vi "PathDrawerMain.vi"() -> ()   [LabVIEW 2020]
uses:
  StartingPositions.ctl
  Dawgma Programming Library/Controls/PurePursuit/PathFileData.ctl
  Dawgma Programming Library/Controls/PurePursuit/RobotNeededPathData.ctl
  <vilib>/Utility/miscctls.llb/LVBoundsTypeDef.ctl
  Robot Project/Configuration/Constants.vi
panel:
  out "Test Inch Coordinates":cluster{dbl, dbl}[](array[cluster])=[{289.544235924933, 135.50670241286863}, {0.0, -0.0}, {328.92225201072387, 121.60857908847186}, {215.42091152815016, 204.99731903485255}, {283.75335120643433, 155.1957104557641}]
  out "value":T1[](array[typedef])=[{"RobotNeeded"={"Path"=[{289.544235924933, 127.39946380697052}, {287.98440012511463, 121.65498051124526}, {286.41922502031144, 115.91988239594286}, {284.8425468097273, 110.20506726948979}, {283.24633395018986, 104.52472200513712}, {281.61937943101464, 98.89861870378402}, {279.9454878089578, 93.35531222737507}, {278.2008591447135, 87.93676042855766}, {276.35024133935286, 82.70511682939853}, {274.3412254828133, 77.75279489984473}, {272.09576087008793, 73.21743176567836}, {269.4975173972782, 69.30417285758647}, {266.3730504540402, 66.31888533561163}, {262.30977093522324, 64.13267492925793}, {257.6170022887625, 62.48225945252617}, {252.50215191030858, 61.19110326109334}, {247.10429046762434, 60.14083593442563}, {241.5166672476604, 59.252088190224804}, {235.8018071548225, 58.471641965553985}, {230.0016338079975, 57.763814107212845}, {224.14425732034206, 57.10467874503091}, {218.2485291335668, 56.478193499430674}, {212.3270758147521, 55.87360015253457}, {206.38842308808773, 55.2836904580848}, {200.43813908174548, 54.70361642727725}, {194.4802433054481, 54.13015590178437}, {188.51708827270537, 53.56111165140166}, {182.55050868849642, 52.99504342054156}, {176.58171996706054, 52.430973067035474}, {170.6114588037997, 51.86824641350337}, {164.6402875329216, 51.306429540500694}, {158.66867548195333, 50.74523633232348}, {152.69698950924862, 50.184482181742624}, {146.72554975069153, 49.62405174097509}, {140.7547236952346, 49.06388019791822}, {134.785000977592, 48.50394578938929}, {128.8170560229984, 47.94426701710933}, {122.8518418626467, 47.38490492824676}, {116.89074159778129, 46.82596881662714}, {110.93580758402727, 46.26763838286973}, {104.99009019888962, 45.7101898480154}, {99.05814276927747, 45.15404369729131}, {93.14674575066984, 44.599832973624785}, {87.26600325213306, 44.04850237548434}, {81.4309817746881, 43.50146179439437}, {75.6641490637674, 42.96081623768789}, {69.99901263505986, 42.429706416458394}, {64.48554690731844, 41.91281674321665}, {59.198284254035755, 41.4171340541128}, {54.24838019418854, 40.953079037223475}, {49.80160857908847, 40.53619302949062}], "MaxVel"=150.0, "MaxAccel"=150.0, "Backwards?"=TRUE, "PointSpacing"=6.0, "LookaheadDist"=17.0, "Speed/Curve"=3.0, "SlowDistanceAtEnd"=0.0, "SlowSpeed"=15.0, "MaxDeAccel"=120.0}, "Meta"={"Path (px)"=[{351, 192}, {336, 249}, {144, 267}], "RobotWidth"=31.5, "RobotLength"=38.5, "CenterOfRotYOffset"=17.0, "Roundedness"=0.8606565656565657, "StartingPositionPreset"=5, "PathName"=""}}, {"RobotNeeded"={"Path"=[{41.694369973190355, 41.694369973190355}, {47.64761218323431, 40.94676925259769}, {53.60085959538599, 40.19914995082028}, {59.554106695902426, 39.451516891020106}, {65.50734952417288, 38.70387941982743}, {71.46058708655964, 37.956246193008944}, {77.41382093064641, 37.2086221311749}, {83.36705361599451, 36.461007989713714}, {89.32028708212145, 35.71340175224902}, {95.27352165286956, 34.96580062830542}, {101.22675591339359, 34.21820267296435}, {107.17998723937053, 33.4706075949886}, {113.13321251833818, 32.723016842705846}, {119.08642860902965, 31.975433361115666}, {125.03963222056859, 31.227861451959267}, {130.99281926364412, 30.480307293161797}, {136.94598341959534, 29.732778542763988}, {142.89911342764645, 28.985292503880892}, {148.8521970948602, 28.237856543424133}, {154.80519717572702, 27.490525695688227}, {160.7580926557246, 26.743311754896478}, {166.7108090144928, 25.996307137451996}, {172.66326246213927, 25.249610988717894}, {178.61533307346468, 24.50335830315379}, {184.56682545232815, 23.757776428670198}, {190.51745097236886, 23.013204152377078}, {196.46678999980696, 22.270130566274368}, {202.4142158693123, 21.529284158414665}, {208.35878682551095, 20.79176138061672}, {214.29909655137962, 20.05920100132194}, {220.23305131995286, 19.334042109666537}, {226.15753100580926, 18.619918062154806}, {232.06788077313638, 17.92224896220281}, {237.95715568369013, 17.249121917891284}, {243.81499755234879, 16.61260080269244}, {249.62595906000692, 16.030669585531108}, {255.36700689486312, 15.530167782478935}, {261.0037825664052, 15.151071217352833}, {266.48505855860725, 14.953090658917299}, {271.7344114271029, 15.025170414334722}, {276.6378873606053, 15.500037107436073}, {281.02552281994616, 16.5756320859188}, {284.64383847846, 18.547123872167777}, {287.2812495218884, 21.833836599641202}, {289.2609081448733, 26.00205669815591}, {290.7994717493821, 30.760784058063827}, {292.04218375653704, 35.914613439968605}, {293.0863889218551, 41.33211000782484}, {293.9972923578865, 46.924534979681674}, {294.8185166544407, 52.63147263946088}, {295.5791655320445, 58.411043001053216}, {296.2985359831856, 64.23312215031287}, {296.9892418555871, 70.074469274851}, {297.6592556133157, 75.91496594399388}, {298.3131992777047, 81.73435754239064}, {298.95309316561156, 87.50897171708034}, {299.57868315910804, 93.20788489320849}, {300.18739942296327, 98.78791642871371}, {300.7739401344564, 104.18663870347694}, {301.32941304122085, 109.31227034681507}, {301.839895859845, 114.02881614064651}, {302.28418230563005, 118.13404825737267}], "MaxVel"=150.0, "MaxAccel"=150.0, "Backwards?"=FALSE, "PointSpacing"=6.0, "LookaheadDist"=17.0, "Speed/Curve"=3.0, "SlowDistanceAtEnd"=0.0, "SlowSpeed"=15.0, "MaxDeAccel"=120.0}, "Meta"={"Path (px)"=[{137, 266}, {352, 293}, {362, 200}], "RobotWidth"=31.5, "RobotLength"=38.5, "CenterOfRotYOffset"=17.0, "Roundedness"=0.8606565656565657, "StartingPositionPreset"=5, "PathName"=""}}] {"RobotNeeded"."SlowSpeed" format="%#_13g"; "RobotNeeded"."SlowDistanceAtEnd" format="%#_13g"; "RobotNeeded"."Speed/Curve" format="%#_13g"}
  in  "NoUpdate":bool
  out "PathsStorage":T1[](array[typedef])=[{"RobotNeeded"={"Path"=[{425.05093833780165, 52.11796246648794}, {430.9905583996291, 52.11796246648794}, {436.9198305935917, 52.11796246648794}, {442.8265331238852, 52.11796246648794}, {448.6941988585669, 52.11796246648794}, {454.50043960617046, 52.11796246648794}, {460.2111611561605, 52.11796246648794}, {465.7769300637667, 52.11796246648794}, {471.1226712041929, 52.11796246648794}, {476.13506368722386, 52.11796246648794}, {480.64343163538877, 52.11796246648794}], "MaxVel"=100.0, "MaxAccel"=150.0, "Backwards?"=FALSE, "PointSpacing"=6.0, "LookaheadDist"=17.0, "Speed/Curve"=3.0, "SlowDistanceAtEnd"=0.0, "SlowSpeed"=15.0, "MaxDeAccel"=120.0}, "Meta"={"Path (px)"=[{468, 257}, {516, 257}], "RobotWidth"=32.0, "RobotLength"=39.0, "CenterOfRotYOffset"=17.0, "Roundedness"=0.8526363636363636, "StartingPositionPreset"=6, "PathName"=""}}] {"RobotNeeded"."SlowSpeed" format="%#_13g"; "RobotNeeded"."SlowDistanceAtEnd" format="%#_13g"; "RobotNeeded"."Speed/Curve" format="%#_13g"}
  in  "Tab Control":enum32{"Path", "Load/Save"}(tab)
  in  "SetStart":bool
  in  "Deaccel":dbl=120.0 format="%#_13g"
  in  "SlowSpeed":dbl=15.0 format="%#_13g"
  in  "SlowDistanceAtEnd":dbl format="%#_13g"
  in  "Speed/Curve":dbl=3.0 format="%#_13g"
  in  "DriveBackwards?":bool
  in  "Lookahead":dbl=17.0
  in  "Points (in)":cluster{dbl, dbl}[](array[cluster])=[{425.05093833780165, 52.11796246648794}, {480.64343163538877, 52.11796246648794}]
  out "Points (px)":cluster{dbl, dbl}[](array[cluster])=[{468.0, 257.0}, {516.0, 257.0}]
  in  "Roundedness":dbl(slide)=0.8526363636363636 scale=0.6..0.997
  in  "PointSpacing":dbl=6.0 min=1.0 format="%#_13g"
  in  "Flip Path":bool
  in  "MaxVel":dbl=100.0 format="%#_13g"
  in  "Accel":dbl=150.0 format="%#_13g"
  in  "StartingPosition":T3=enum."No Preset"
  in  "Multiple Paths":i32(listbox)
  in  "ExportAllToRobot":bool
  in  "LocalTempPaths":i32(listbox)
  out "standard output":string
  in  "SaveToLocal":bool
  in  "LoadFromLocal":bool
  in  "ExportToRobot":bool
  in  "LoadAllFromRobot":bool
  in  "LocalPaths":i32(listbox)
  out "standard error":string="NI Linux Real-Time (run mode)\n\nLog in with your NI-Auth credentials.\n\n"
  in  "LocalFileNames":string[](array[string])=["STARTINGPOSITIONTEST.txt"]
  out "Path Drawer":T4(plugin-control)
  # "(Double Click)"
  # "INSTRUCTIONS"
  # "The red line is the path that the robot recieves. Everything else is to help create that path\n\nUse the multi-line tool to draw a path. Double click to stop drawing.\nHover over a node and press backspace to remove it.\nPress I to insert a new node (at the end of the path only, for now)\n\nUse the contols to input robot width, height, and center of rotation offset,\nHow far apart the points in the \"real world units\" path are,\nWhether the robot travels on the left or right of your green lines, and\nthe roundedness of the path. (Note: point spacing affects roundedness)\n\nYou can manually edit the green node's location in the path with the Points array,\nor drag the nodes on the image\n\nPress Export To File and enter the file name (no extension) to save the path to a file in the\nThisVIsDirectory\\Paths\\ folder\n\nIf you acidentally clear your path press Z quickly to get it back"
  # "Responses of CMDs run"
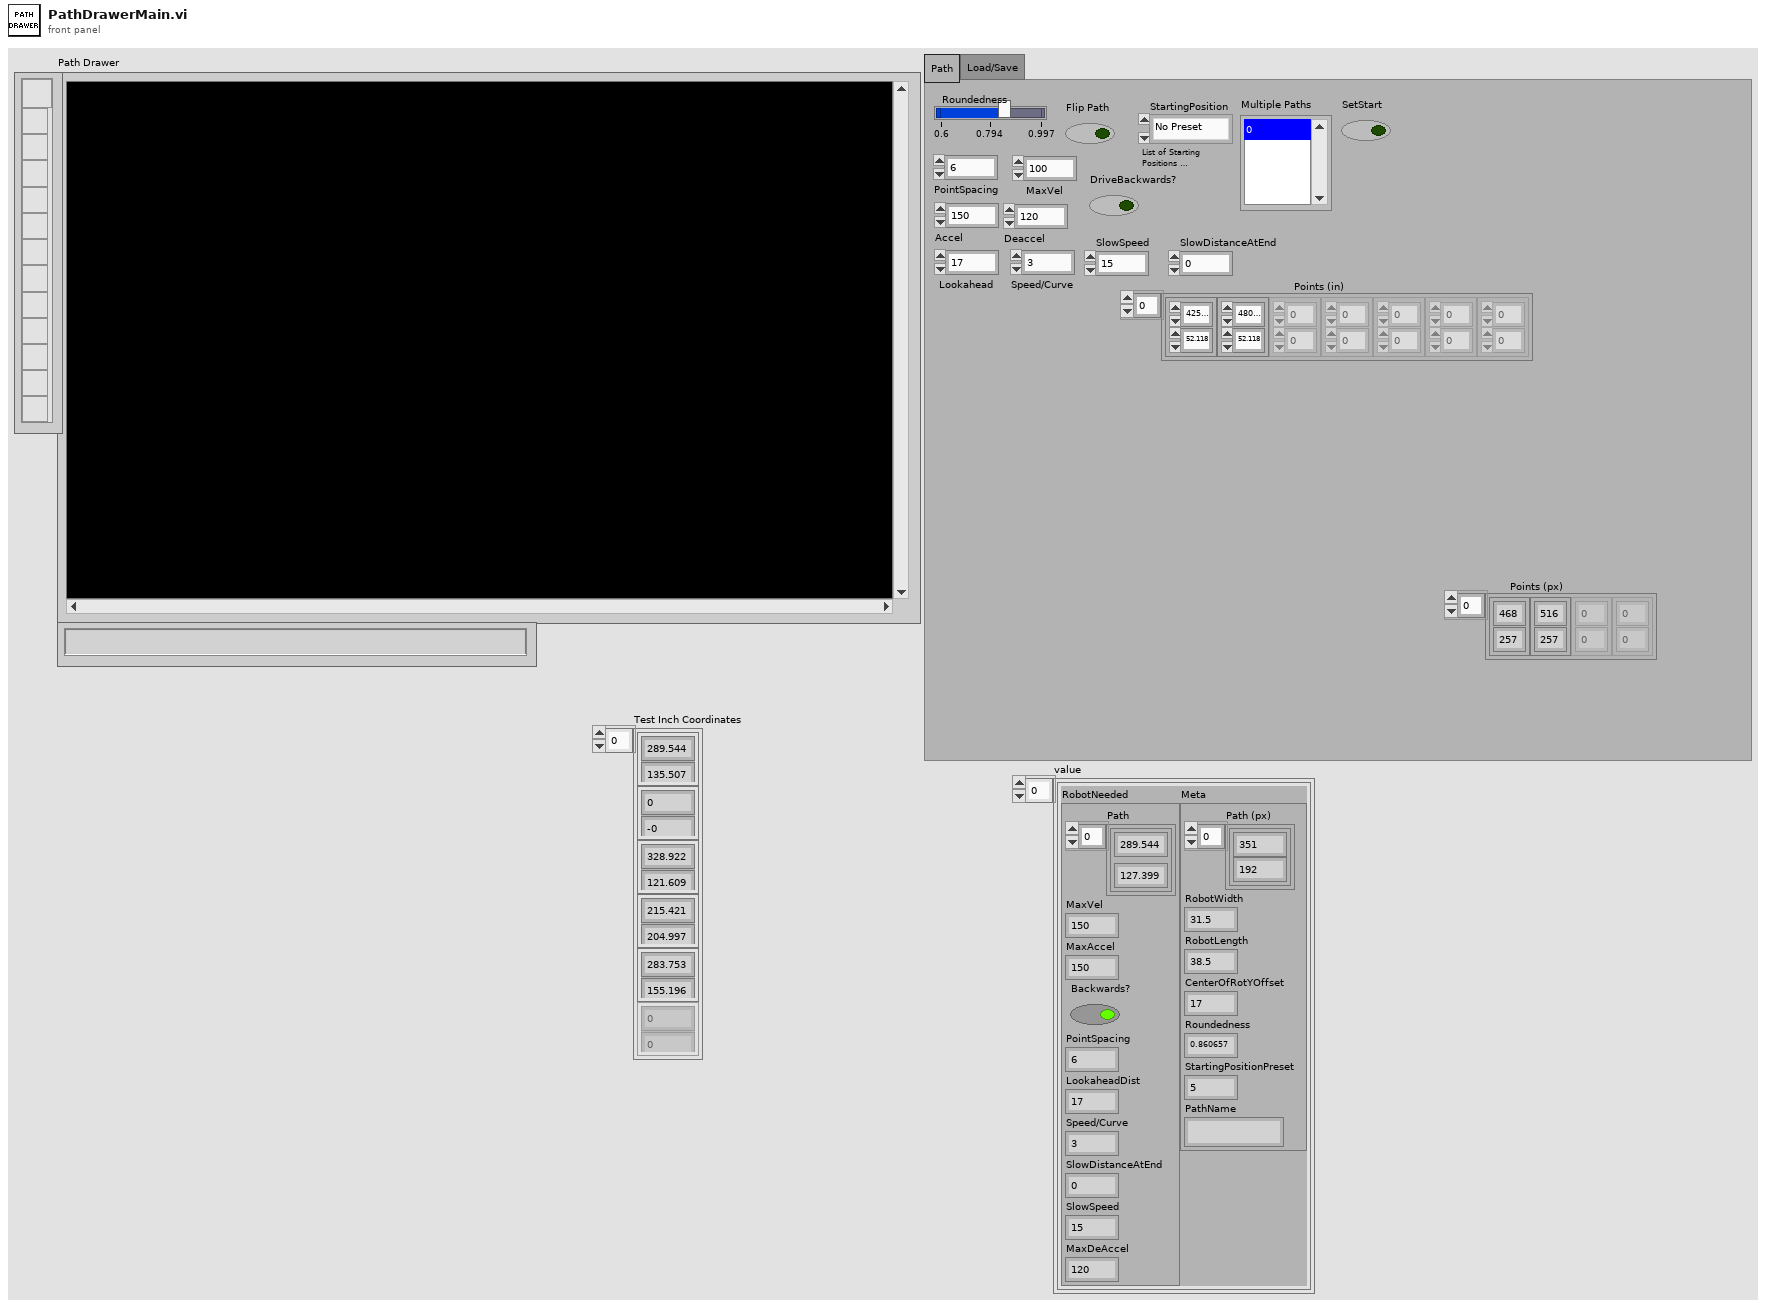
[diagram p1: front panel]
types:
  T1 = typedef "PathFileData.ctl" = cluster{"RobotNeeded":T2, "Meta":cluster{"Path (px)":cluster{i32, i32}[], "RobotWidth":dbl, "RobotLength":dbl, "CenterOfRotYOffset":dbl, "Roundedness":dbl, "StartingPositionPreset":u32, "PathName":string}}
  T2 = typedef "RobotNeededPathData.ctl" = cluster{"Path":cluster{dbl, dbl}[], "MaxVel":dbl, "MaxAccel":dbl, "Backwards?":bool, "PointSpacing":dbl, "LookaheadDist":dbl, "Speed/Curve":dbl, "SlowDistanceAtEnd":dbl, "SlowSpeed":dbl, "MaxDeAccel":dbl}
  T3 = typedef "StartingPositions.ctl" = enum16{"1", "2", "3", "4", "5", "6", "No Preset"}
  T4 = typedef "IMAQ Image.ctl" = refnum<image>
  T5 = typedef "Image Type" = u32
  T6 = enum16{"open", "replace", "create", "open or create", "replace or create", "replace or create with confirmation"}
  T7 = typedef "LVBoundsTypeDef.ctl" = cluster{"Width":u32, "Height":u32}
  T8 = cluster{"Global Rectangle":i32[], "Contours":cluster{"Contour Type":u32, "ROI Type":u32, "Points":i32[]}[]}
  T9 = cluster{"Contour Type":u32, "ROI Type":u32, "Points":i32[]}[]
  T10 = cluster{"Contour Type":u32, "ROI Type":u32, "Points":i32[]}
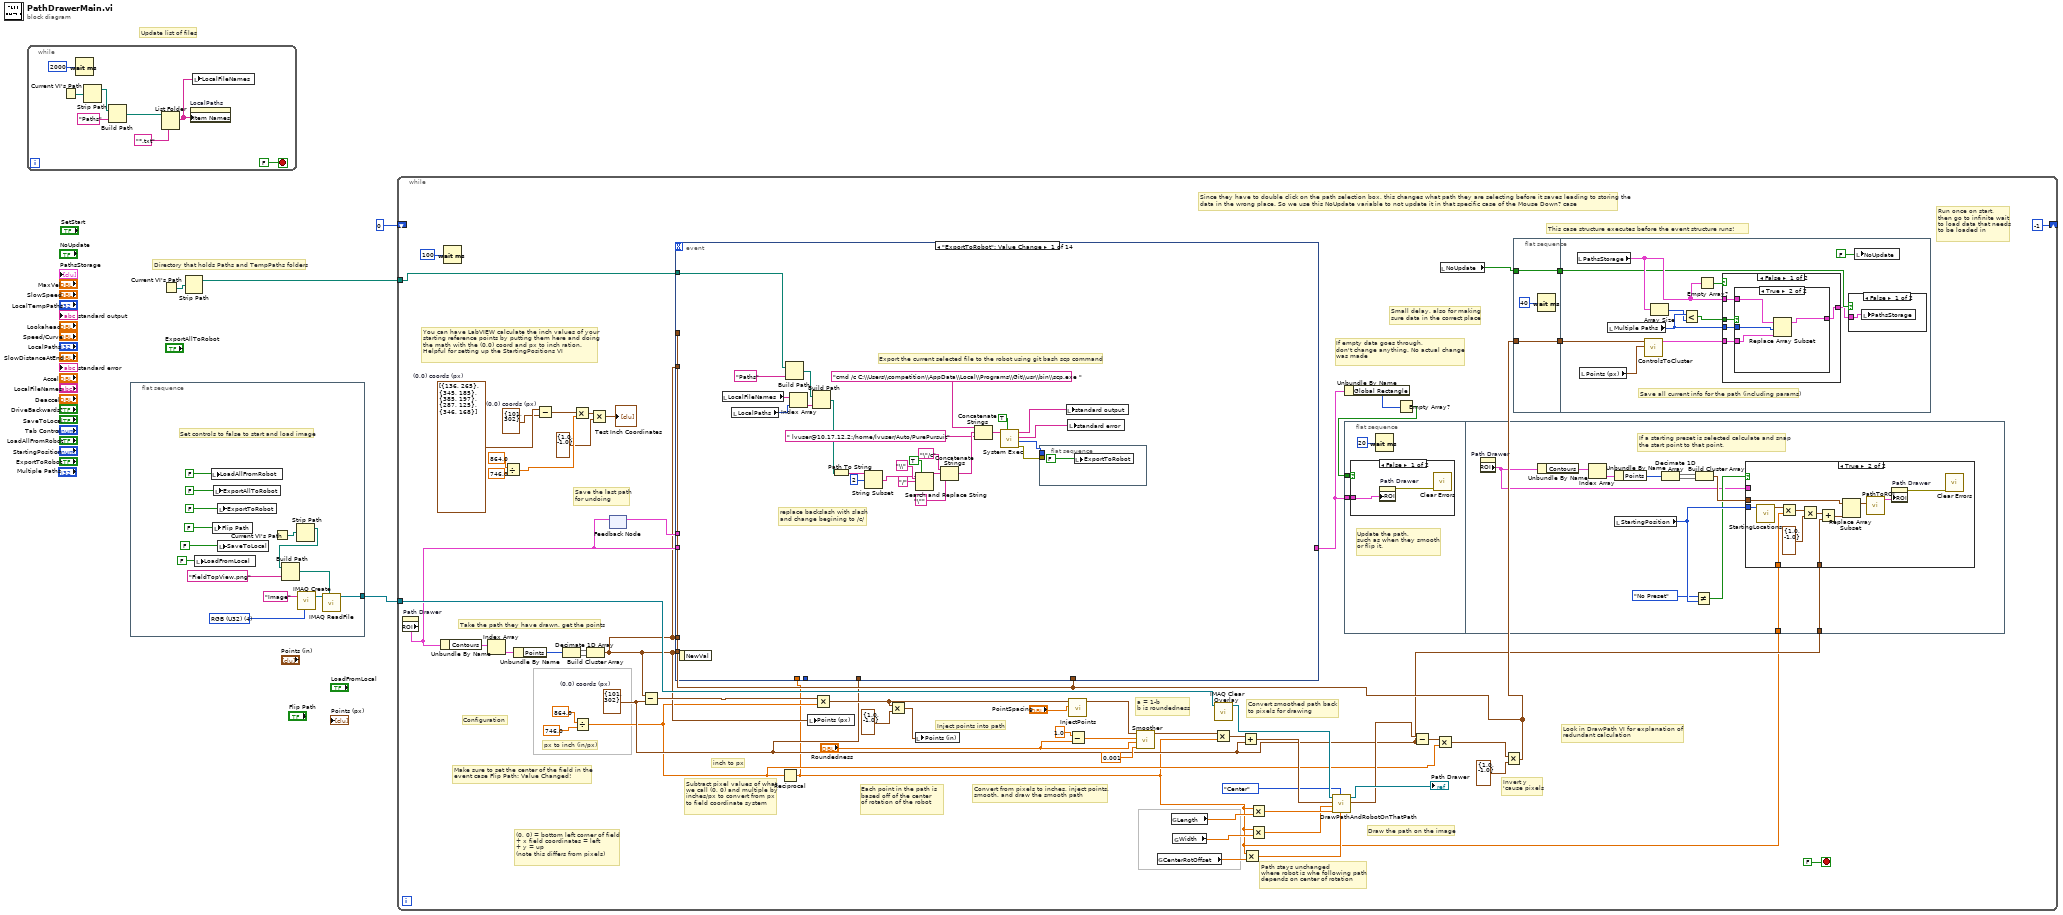
[diagram p0: block diagram]
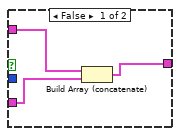
[diagram p3: hidden frame]
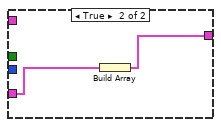
[diagram p4: hidden frame]
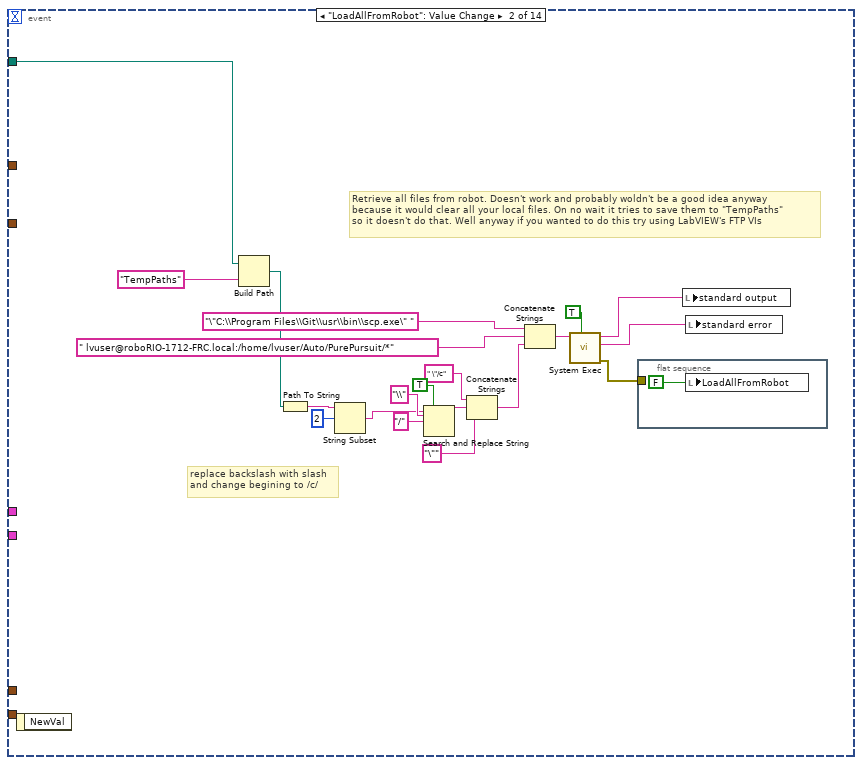
[diagram p7: hidden frame]
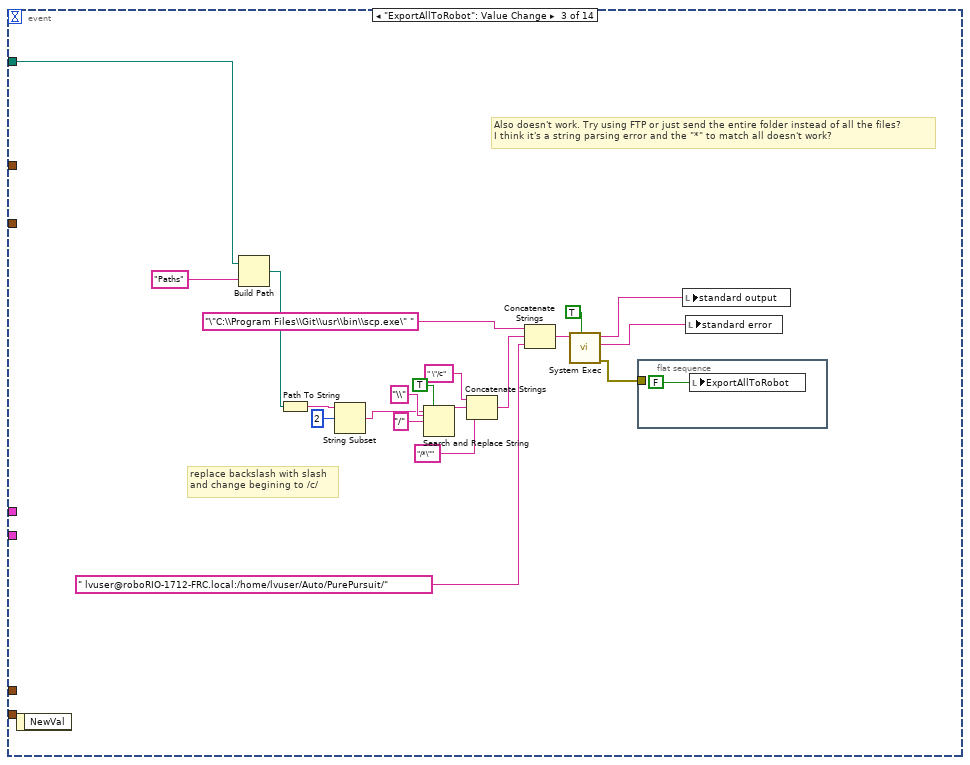
[diagram p8: hidden frame]
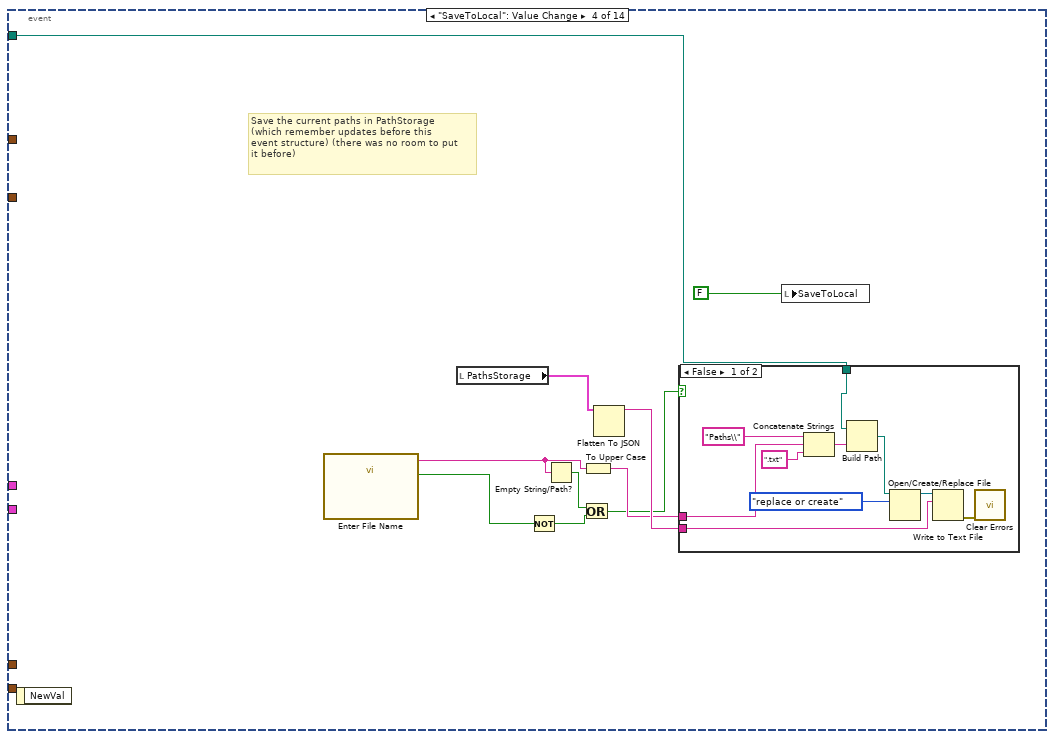
[diagram p9: hidden frame]
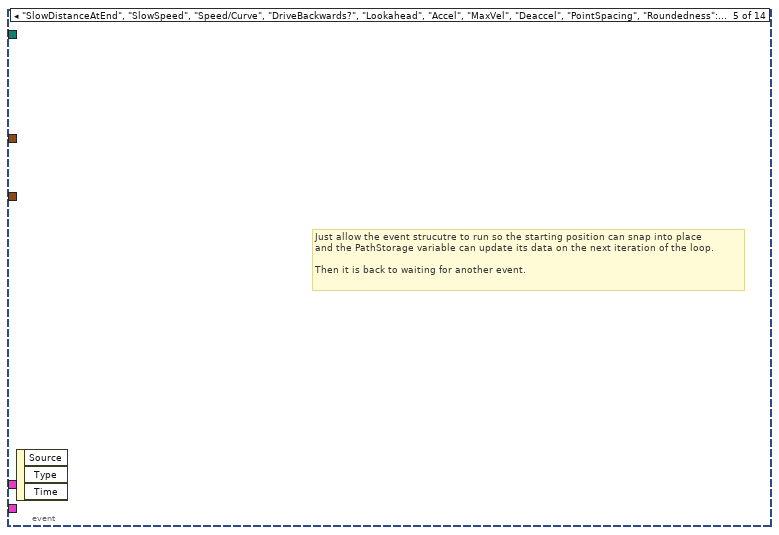
[diagram p11: hidden frame]
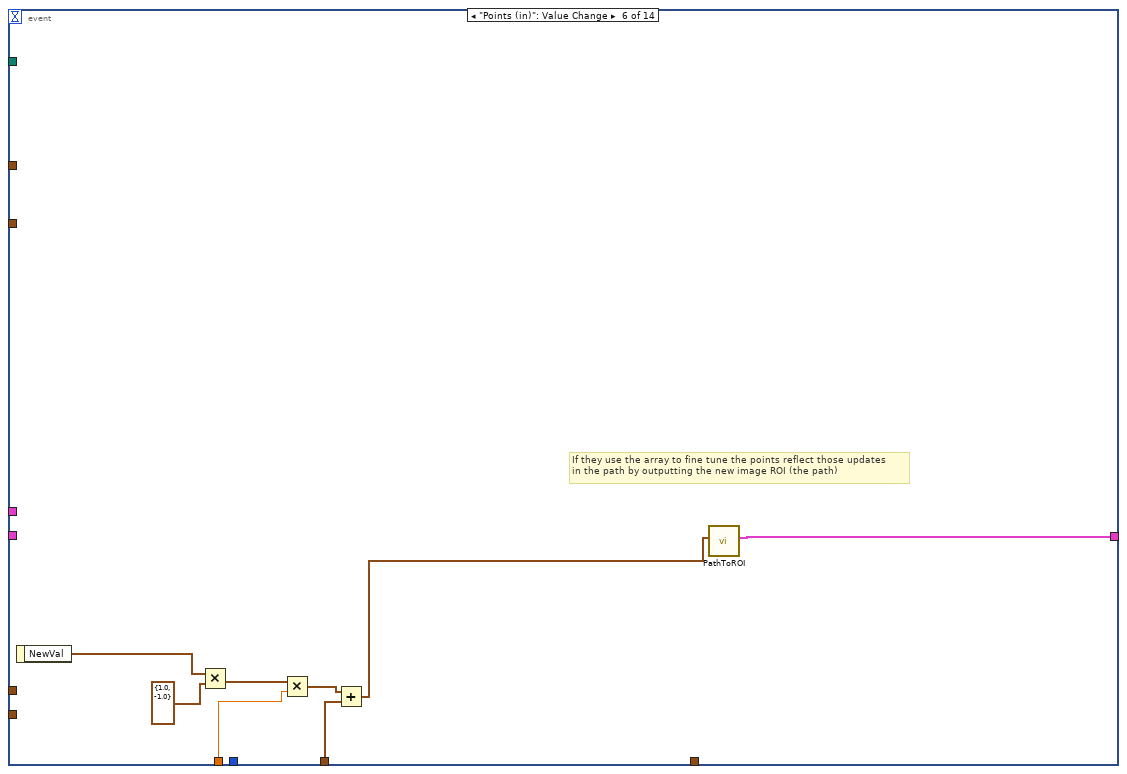
[diagram p12: hidden frame]
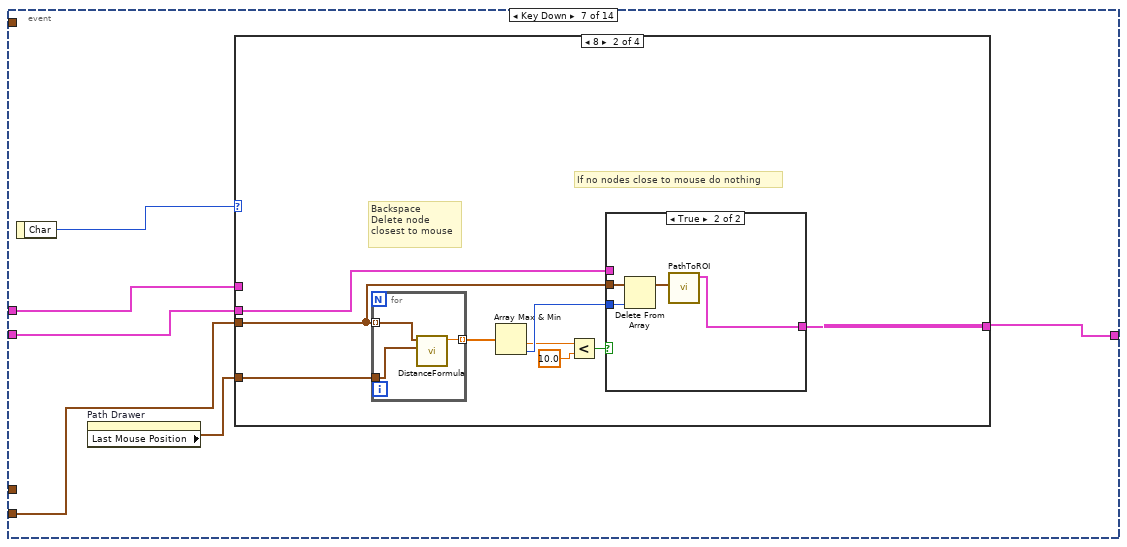
[diagram p13: hidden frame]
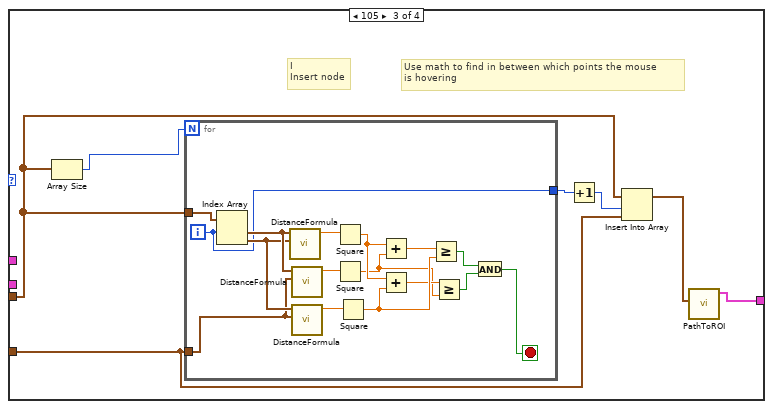
[diagram p16: hidden frame]
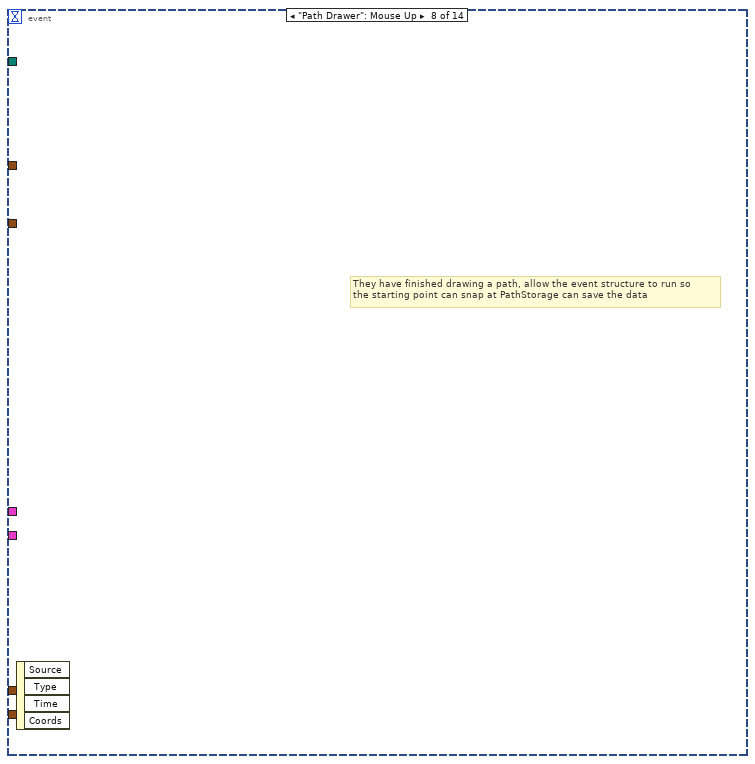
[diagram p18: hidden frame]
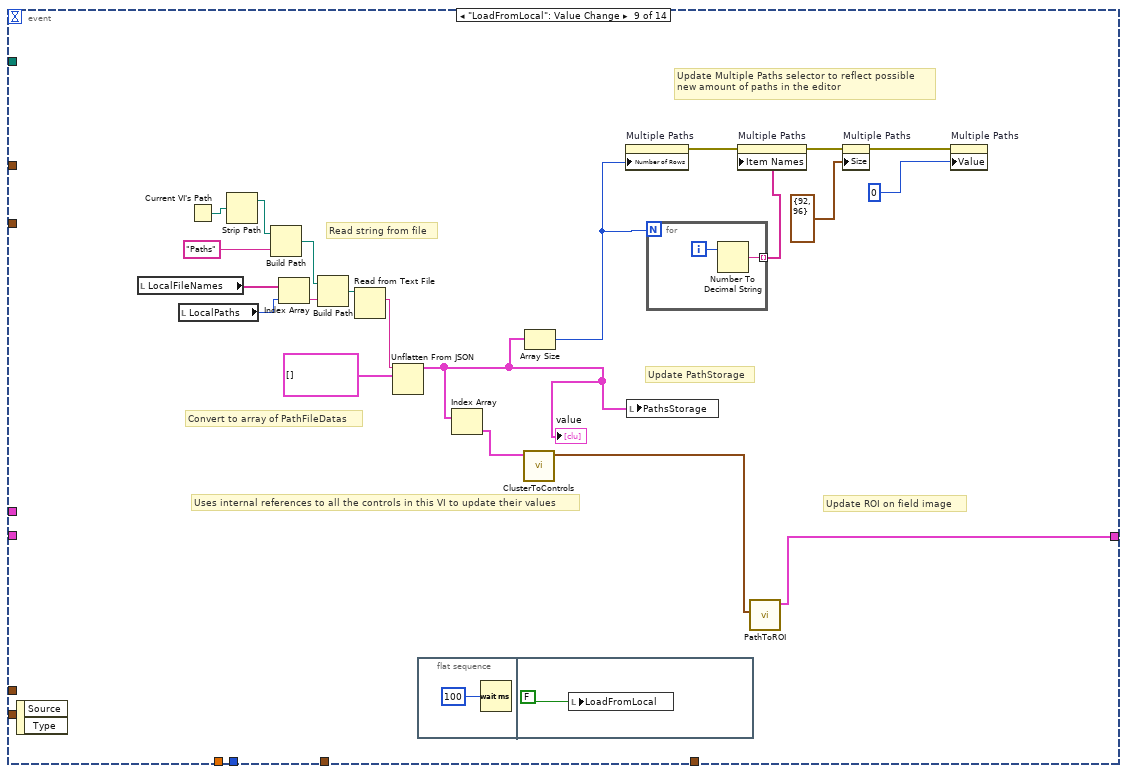
[diagram p19: hidden frame]
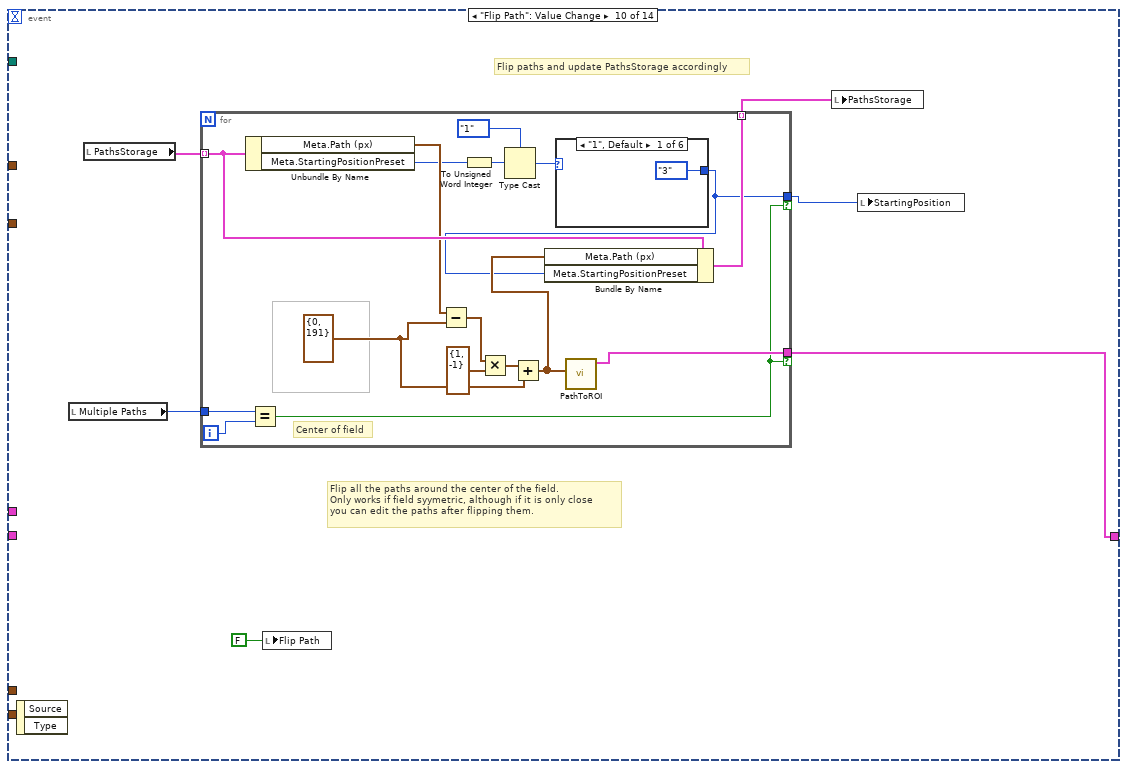
[diagram p20: hidden frame]
diagram:
  # "Update list of files"
  # "Directory that holds Paths and TempPaths folders"
  n1 = while {
    stop <- FALSE stop-if-true
    n2 = Current VI's Path() -> (path=w7:path)
    n3 = Wait (ms)(milliseconds to wait=u32 2000) -> ()  [unwired: 1 out]
    n4 = Strip Path(path=w7) -> (stripped path=w6:path)  [unwired: 1 out]
    n5 = Build Path(base path=w6, name or relative path="Paths") -> (appended path=w9:path)
    n6 = List Folder(path=w9, pattern="*.txt") -> (filenames=w11:string[])  [unwired: 2 in, 3 out]
    n7 = property on="LocalPaths" class="LstBox (strict)"("Item Names"=w11) -> ()  [unwired: 2 in, 2 out]
    n8 = local write "LocalFileNames"(w11) -> ()
  }
  n9 = flat-sequence {
    tunnel: [w21] -> w4
    frame #0 {
      w23 = T5 4 items=["Grayscale (U8)", "Grayscale (I16)", "Grayscale (SGL)", "Complex (CSG)", "RGB (U32)", "HSL (U32)", "RGB (U64)", "Grayscale (U16)"] ("Image Type")
      # "Set controls to false to start and load image"
      n10 = local write "LoadFromLocal"(FALSE ("Export To File")) -> ()
      n11 = local write "LoadAllFromRobot"(FALSE ("Export To File")) -> ()
      n12 = local write "Flip Path"(FALSE ("Export To File")) -> ()
      n13 = local write "ExportAllToRobot"(FALSE ("Export To File")) -> ()
      n14 = local write "ExportToRobot"(FALSE ("Export To File")) -> ()
      n15 = local write "SaveToLocal"(FALSE ("Export To File")) -> ()
      n16 = Current VI's Path() -> (path=w16:path)
      n17 = Strip Path(path=w16) -> (stripped path=w15:path)  [unwired: 1 out]
      n18 = Build Path(base path=w15, name or relative path="FieldTopView.png") -> (appended path=w25:path)
      n19 = call "IMAQ Create"("Image Name"="Image", "Image Type"=w23) -> ("New Image"=w22:T4)  [unwired: 3 in, 1 out]
      n20 = call "IMAQ ReadFile"("File Path"=w25, "Image"=w22) -> ("Image Out"=w21:T4)  [unwired: 5 in, 4 out]
    }
  }
  n21 = Current VI's Path() -> (path=w3:path)
  n22 = Strip Path(path=w3) -> (stripped path=w2:path)  [unwired: 1 out]
  n23 = while {
    tunnel: w4 -> [w80]
    tunnel: w2 -> [w55]
    shift-right: [-1] -> _
    shift-left: 0 -> [_]
    stop <- FALSE stop-if-true
    w27 = cluster{i32, i32} {101, 302}  # (0,0) coords (px)
    w28 = cluster{i32, i32}[] [{136, 265}, {345, 185}, {385, 197}, {287, 125}, {346, 168}]  # (0,0) coords (px)
    w38 = cluster{i32, i32} {101, 302}  # (0,0) coords (px)
    # "Each point in the path is\nbased off of the center\nof rotation of the robot"
    # "You can have LabVIEW calculate the inch values of your\nstarting reference points by putting them here and doing\nthe math with the (0,0) coord and px to inch ration.\nHelpful for setting up the StartingPositions VI"
    # "Small delay, also for making\nsure data in the correct place"
    # "Since they have to double click on the path selection box, this changes what path they are selecting before it saves leading to storing the\ndata in the wrong place. So we use this NoUpdate variable to not update it in that specific case of the Mouse Down? case"
    # "This case structure executes before the event structure runs!"
    # "Look in DrawPath VI for explanation of \nredundant calculation"
    # "Draw the path on the image"
    # "a = 1-b\nb is roundedness"
    # "Inject points into path"
    # "(0, 0) = bottom left corner of field\n+ x field coordinates = left\n+ y = up\n(note this differs from pixels)"
    # "Take the path they have drawn, get the points"
    # "Save the last path\nfor undoing"
    # "Make sure to set the center of the field in the\nevent case Flip Path: Value Changed!"
    # "inch to px"
    # "px to inch (in/px)"
    # "Configuration"
    # "Run once on start,\nthen go to infinite wait\nto load data that needs\nto be loaded in"
    # "Invert y\n'cause pixels"
    # "Path stays unchanged\nwhere robot is whe following path\ndepends on center of rotation"
    # "Convert smoothed path back\nto pixels for drawing"
    # "If empty data goes through,\ndon't change anything. No actual change\nwas made"
    # "Convert from pixels to inches, inject points,\nsmooth, and draw the smooth path"
    # "Subtract pixel values of what\nwe call (0, 0) and multiple by\ninches/px to convert from px\nto field coordinate system"
    n24 = property on="Path Drawer" class="ImageControl"() -> ("ROI"=w57:T8)  [unwired: 2 in, 2 out]
    n25 = Unbundle By Name(w57) -> ("Contours"=w86:T9)
    n26 = Wait (ms)(milliseconds to wait=u32 100) -> ()  [unwired: 1 out]
    n27 = Index Array(array=w86) -> (element=w81:T10)  [unwired: 1 in]
    n28 = Divide(x=864.0, y=746.0) -> (x/y=w32:dbl)
    n29 = Unbundle By Name(w81) -> ("Points"=w75:i32[])
    n30 = Subtract(x=w28, y=w27) -> (x-y=w33:cluster{i32, i32}[])
    n31 = Decimate 1D Array(w75) -> (w85:i32[], w84:i32[])
    n32 = Multiply(x=w33, y=w32) -> (x*y=w31:cluster{dbl, dbl}[])
    n33 = Divide(x=864.0, y=746.0) -> (x/y=w37:dbl)
    n34 = Build Cluster Array(w85, w84) -> (w42:cluster{i32, i32}[])
    n35 = Multiply(x=w31, y=cluster{dbl, dbl} {1.0, -1.0}) -> (x*y=→"Test Inch Coordinates":cluster{dbl, dbl}[])
    n36 = feedback-in #1(w57) -> ()
    n37 = feedback #1() -> (w67:T8)  [unwired: 1 in]
    n38 = Subtract(x=w42, y=w38) -> (x-y=w76:cluster{i32, i32}[])
    n39 = Reciprocal(x=w37) -> (1/x=w36:dbl)
    n40 = local write "Points (px)"(w42) -> ()
    n41 = Multiply(x=w76, y=w37) -> (x*y=w40:cluster{dbl, dbl}[])
    n42 = Multiply(x=w40, y=cluster{dbl, dbl} {1.0, -1.0}) -> (x*y=w39:cluster{dbl, dbl}[])
    n43 = local write "Points (in)"(w39) -> ()
    n44 = call "InjectPoints.vi"("Distance"="PointSpacing", "Path"=w40) -> ("Path out"=w78:cluster{dbl, dbl}[])  [unwired: 9 in]
    n45 = Subtract(x=1.0, y="Roundedness") -> (x-y=w73:dbl)
    n46 = call "Smoother.vi"("tolerance"=0.001, "B"="Roundedness", "A"=w73, "Path"=w78) -> ("SmoothPath"=w69:cluster{dbl, dbl}[])  [unwired: 7 in]
    n47 = global read "Constants.vi" "CenterRotOffset"() -> (w43:dbl)
    n48 = global read "Constants.vi" "Length"() -> (w45:dbl)
    n49 = global read "Constants.vi" "Width"() -> (w44:dbl)
    n50 = Multiply(x=w69, y=w36) -> (x*y=w77:cluster{dbl, dbl}[])
    n51 = call "IMAQ Clear Overlay"("Image"=w80) -> ("Image Out"=w63:T4)  [unwired: 9 in, 1 out]
    n52 = Add(x=w77, y=w38) -> (x+y=w62:cluster{dbl, dbl}[])
    n53 = Multiply(x=w36, y=w43) -> (x*y=w52:dbl)
    n54 = Multiply(x=w36, y=w45) -> (x*y=w61:dbl)
    n55 = Multiply(x=w36, y=w44) -> (x*y=w53:dbl)
    n56 = call "DrawPathAndRobotOnThatPath.vi"("CenterOfRotYOffset (px)"=w52, "PathMode"=enum16{"Left", "Right", "Center"}."Center", "RobotLength (px)"=w61, "RobotWidth (px)"=w53, "Path (px)"=w62, "Image In"=w63) -> ("NewPath (px)"=w64:cluster{dbl, dbl}[], "Image Out"=→"Path Drawer":T4)  [unwired: 4 in]
    n57 = flat-sequence {
      tunnel: w56 -> [w118]
      tunnel: w54 -> [w117]
      tunnel: w36 -> [w123]
      tunnel: w38 -> [w122]
      frame #0 {
        # "Update the path,\nsuch as when they smooth\nor flip it."
        n58 = case shown="False" w117 {
          tunnel: w118 -> [w119 _]
          frame False {
            n59 = property on="Path Drawer" class="ImageControl"("ROI"=w119) -> (error out=w120:errorcluster)  [unwired: 2 in, 1 out]
            n60 = call <vilib>:"Clear Errors.vi"("error in (no error)"=w120) -> ()  [unwired: 5 in, 2 out]
          }
          frame True {
          }
        }
        n61 = Wait (ms)(milliseconds to wait=u32 20) -> ()  [unwired: 1 out]
      }
      frame #1 {
        # "If a starting preset is selected calculate and snap\nthe start point to that point."
        n62 = property on="Path Drawer" class="ImageControl"() -> ("ROI"=w124:T8)  [unwired: 2 in, 2 out]
        n63 = Unbundle By Name(w124) -> ("Contours"=w127:T9)
        n64 = Index Array(array=w127) -> (element=w130:T10)  [unwired: 1 in]
        n65 = Unbundle By Name(w130) -> ("Points"=w131:i32[])
        n66 = local read "StartingPosition"() -> (w132:T3)
        n67 = Decimate 1D Array(w131) -> (w128:i32[], w129:i32[])
        n68 = Not Equal?(x=StartingPositions."No Preset" ("StartingPosition"), y=w132) -> (x != y?=w125:bool)
        n69 = Build Cluster Array(w128, w129) -> (w126:cluster{i32, i32}[])
        n70 = case shown="True" w125 {
          tunnel: w124 -> [_ _]
          tunnel: w126 -> [_ w143]
          tunnel: w132 -> [_ w133]
          tunnel: w123 -> [_ w139]
          tunnel: w122 -> [_ w137]
          frame False {
          }
          frame True {
            n71 = call "StartingLocations.vi"("Index"=w133) -> ("Location"=w140:cluster{dbl, dbl})  [unwired: 10 in]
            n72 = Multiply(x=w140, y=w139) -> (x*y=w136:cluster{dbl, dbl})
            n73 = Multiply(x=w136, y=cluster{dbl, dbl} {1.0, -1.0}) -> (x*y=w134:cluster{dbl, dbl})
            n74 = Add(x=w134, y=w137) -> (x+y=w138:cluster{dbl, dbl})
            n75 = Replace Array Subset(array=w143, new element=w138) -> (w144:cluster{i32, i32}[])  [unwired: 1 in]
            n76 = call "PathToROI.vi"("Path In"=w144) -> ("ROI Out"=w141:T8)  [unwired: 10 in]
            n77 = property on="Path Drawer" class="ImageControl"("ROI"=w141) -> (error out=w142:errorcluster)  [unwired: 2 in, 1 out]
            n78 = call <vilib>:"Clear Errors.vi"("error in (no error)"=w142) -> ()  [unwired: 5 in, 2 out]
          }
        }
      }
    }
    n79 = Subtract(x=w64, y=w38) -> (x-y=w68:cluster{dbl, dbl}[])
    n80 = Multiply(x=w68, y=w37) -> (x*y=w59:cluster{dbl, dbl}[])
    n81 = local read "NoUpdate"() -> (w46:bool)
    n82 = Multiply(x=w59, y=cluster{dbl, dbl} {1.0, -1.0}) -> (x*y=w49:cluster{dbl, dbl}[])
    n83 = event shown="[0] \"ExportToRobot\": Value Change" {
      selector: _ -> [_ _ _ _ _ _ _ _ _ _ _ _ _ _]
      dyn-events: _ -> [_ _ _ _ _ _ _ _ _ _ _ _ _ _]
      timeout: _ -> [_ _ _ _ _ _ _ _ _ _ _ _ _ _]
      tunnel: w57 -> [_ _ _ _ _ _ w246 _ _ _ _ _ w356 w417]
      tunnel: [_ _ _ _ _ w240 w243 _ w308 w317 w344 _ w355 w418] -> w56
      tunnel: w49 -> [_ _ _ _ _ _ _ _ _ _ _ _ _ _]
      tunnel: w67 -> [_ _ _ _ _ _ w242 _ _ _ _ _ _ _]
      tunnel: w42 -> [_ _ _ _ _ _ w241 _ _ _ _ _ _ _]
      tunnel: w42 -> [_ _ _ _ _ _ _ _ _ _ _ _ _ _]
      tunnel: w49 -> [_ _ _ _ _ _ _ _ _ _ _ _ _ _]
      tunnel: w55 -> [w150 w171 w192 w215 _ _ _ _ _ _ _ _ _ _]
      tunnel: [_ _ _ _ _ _ _ _ _ _ w343 _ _ _] -> _
      tunnel: w42 -> [_ _ _ _ _ _ _ _ _ _ _ _ _ _]
      tunnel: w36 -> [_ _ _ _ _ w237 _ _ _ _ _ _ _ _]
      tunnel: w38 -> [_ _ _ _ _ w234 _ _ _ _ _ _ _ _]
      event "ExportToRobot": Value Change {
        # "Export the current selected file to the robot using git bash scp command"
        # "replace backslash with slash\nand change begining to /c/"
        n84 = event-data() -> ()  [unwired: 1 in, 1 out]
        n85 = local read "LocalFileNames"() -> (w157:string[])
        n86 = local read "LocalPaths"() -> (w158:i32)
        n87 = Build Path(base path=w150, name or relative path="Paths") -> (appended path=w159:path)
        n88 = Index Array(array=w157, index=w158) -> (element=w148:string)
        n89 = Build Path(base path=w159, name or relative path=w148) -> (appended path=w155:path)
        n90 = Path To String(path=w155) -> (string=w164:string)
        n91 = String Subset(string=w164, offset (0)=2) -> (substring=w162:string)  [unwired: 1 in]
        n92 = Search and Replace String(replace all?=TRUE ("replace all? (F)"), input string=w162, search string="\\", replace string="/" ("replace string (\"\")")) -> (result string=w161:string)  [unwired: 4 in, 3 out]
        n93 = Concatenate Strings("\"/c" ("string"), w161, "\"" ("string")) -> (w146:string)
        n94 = Concatenate Strings("cmd /c C:\\Users\\competition\\AppData\\Local\\Programs\\Git\\usr\\bin\\scp.exe " ("command line"), w146, " lvuser@10.17.12.2:/home/lvuser/Auto/PurePursuit" ("string")) -> (w168:string)
        n95 = call <vilib>:"System Exec.vi"("wait until completion? (T)"=TRUE, "command line"=w168) -> ("error out"=w153:errorcluster, "return code"=w149:i32, "standard error"=w151:string, "standard output"=w152:string)  [unwired: 6 in]
        n96 = flat-sequence {
          tunnel: w153 -> [_]
          tunnel: w149 -> [_]
          frame #0 {
            n97 = local write "ExportToRobot"(FALSE ("Export To File")) -> ()
          }
        }
        n98 = local write "standard output"(w152) -> ()
        n99 = local write "standard error"(w151) -> ()
      }
      event "LoadAllFromRobot": Value Change {
        # "Retrieve all files from robot. Doesn't work and probably woldn't be a good idea anyway\nbecause it would clear all your local files. On no wait it tries to save them to \"TempPaths\"\nso it doesn't do that. Well anyway if you wanted to do this try using LabVIEW's FTP VIs"
        # "replace backslash with slash\nand change begining to /c/"
        n100 = event-data() -> ()  [unwired: 1 in, 1 out]
        n101 = Build Path(base path=w171, name or relative path="TempPaths") -> (appended path=w174:path)
        n102 = Path To String(path=w174) -> (string=w184:string)
        n103 = String Subset(string=w184, offset (0)=2) -> (substring=w182:string)  [unwired: 1 in]
        n104 = Search and Replace String(replace all?=TRUE ("replace all? (F)"), input string=w182, search string="\\", replace string="/" ("replace string (\"\")")) -> (result string=w181:string)  [unwired: 4 in, 3 out]
        n105 = Concatenate Strings(" \"/c" ("string"), w181, "\"" ("string")) -> (w172:string)
        n106 = Concatenate Strings("\"C:\\Program Files\\Git\\usr\\bin\\scp.exe\" " ("command line"), " lvuser@roboRIO-1712-FRC.local:/home/lvuser/Auto/PurePursuit/*" ("string"), w172) -> (w188:string)
        n107 = call <vilib>:"System Exec.vi"("wait until completion? (T)"=TRUE, "command line"=w188) -> ("error out"=w177:errorcluster, "standard error"=w175:string, "standard output"=w176:string)  [unwired: 6 in, 1 out]
        n108 = flat-sequence {
          tunnel: w177 -> [_]
          frame #0 {
            n109 = local write "LoadAllFromRobot"(FALSE ("Export To File")) -> ()
          }
        }
        n110 = local write "standard output"(w176) -> ()
        n111 = local write "standard error"(w175) -> ()
      }
      event "ExportAllToRobot": Value Change {
        # "Also doesn't work. Try using FTP or just send the entire folder instead of all the files?\nI think it's a string parsing error and the \"*\" to match all doesn't work?"
        # "replace backslash with slash\nand change begining to /c/"
        n112 = event-data() -> ()  [unwired: 1 in, 1 out]
        n113 = Build Path(base path=w192, name or relative path="Paths") -> (appended path=w195:path)
        n114 = Path To String(path=w195) -> (string=w205:string)
        n115 = String Subset(string=w205, offset (0)=2) -> (substring=w203:string)  [unwired: 1 in]
        n116 = Search and Replace String(replace all?=TRUE ("replace all? (F)"), input string=w203, search string="\\", replace string="/" ("replace string (\"\")")) -> (result string=w202:string)  [unwired: 4 in, 3 out]
        n117 = Concatenate Strings(" \"/c" ("string"), w202, "/*\"" ("string")) -> (w194:string)
        n118 = Concatenate Strings("\"C:\\Program Files\\Git\\usr\\bin\\scp.exe\" " ("command line"), w194, " lvuser@roboRIO-1712-FRC.local:/home/lvuser/Auto/PurePursuit/" ("string")) -> (w209:string)
        n119 = call <vilib>:"System Exec.vi"("wait until completion? (T)"=TRUE, "command line"=w209) -> ("error out"=w198:errorcluster, "standard error"=w196:string, "standard output"=w197:string)  [unwired: 6 in, 1 out]
        n120 = flat-sequence {
          tunnel: w198 -> [_]
          frame #0 {
            n121 = local write "ExportAllToRobot"(FALSE ("Export To File")) -> ()
          }
        }
        n122 = local write "standard output"(w197) -> ()
        n123 = local write "standard error"(w196) -> ()
      }
      event "SaveToLocal": Value Change {
        # "Save the current paths in PathStorage\n(which remember updates before this\nevent structure) (there was no room to put\nit before)"
        n124 = event-data() -> ()  [unwired: 1 in, 1 out]
        n125 = call "Enter File Name"() -> ("File Name"=w217:string, "Enter"=w219:bool)  [unwired: 17 in, 1 out]
        n126 = local read "PathsStorage"() -> (w213:T1[])
        n127 = Not(x=w219) -> (.not. x?=w218:bool)
        n128 = Empty String/Path?(string/path=w217) -> (empty?=w220:bool)
        n129 = Or(x=w220, y=w218) -> (x .or. y?=w214:bool)
        n130 = To Upper Case(1:w217) -> (0:w216:string)
        n131 = Flatten To JSON(anything=w213) -> (JSON string=w221:string)  [unwired: 2 in, 1 out]
        n132 = case shown="False" w214 {
          tunnel: w216 -> [w228 _]
          tunnel: w221 -> [w227 _]
          tunnel: w215 -> [w223 _]
          frame False {
            n133 = Concatenate Strings("Paths\\" ("name or relative path"), w228, ".txt" ("string")) -> (w232:string)
            n134 = Build Path(base path=w223, name or relative path=w232) -> (appended path=w226:path)
            n135 = Open/Create/Replace File(file path (use dialog)=w226, operation (0:open)=T6."replace or create") -> (refnum out=w225:refnum<file>)  [unwired: 4 in, 2 out]
            n136 = Write to Text File(file (use dialog)=w225, text=w227) -> (error out=w230:errorcluster)  [unwired: 2 in, 2 out]
            n137 = call <vilib>:"Clear Errors.vi"("error in (no error)"=w230) -> ()  [unwired: 5 in, 2 out]
          }
          frame True {
          }
        }
        n138 = local write "SaveToLocal"(FALSE ("Export To File")) -> ()
      }
      event "SlowDistanceAtEnd", "SlowSpeed", "Speed/Curve", "DriveBackwards?", "Lookahead", "Accel", "MaxVel", "Deaccel", "PointSpacing", "Roundedness": Value Change; Mouse Down; Timeout {
        # "Just allow the event strucutre to run so the starting position can snap into place\nand the PathStorage variable can update its data on the next iteration of the loop.\n\nThen it is back to waiting for another event."
        n139 = event-data() -> ()  [unwired: 1 in, 3 out]
      }
      event "Points (in)": Value Change {
        # "If they use the array to fine tune the points reflect those updates\nin the path by outputting the new image ROI (the path)"
        n140 = event-data() -> ("NewVal"=w238:cluster{dbl, dbl}[])  [unwired: 1 in]
        n141 = Multiply(x=w238, y=cluster{dbl, dbl} {1.0, -1.0}) -> (x*y=w236:cluster{dbl, dbl}[])
        n142 = Multiply(x=w236, y=w237) -> (x*y=w235:cluster{dbl, dbl}[])
        n143 = Add(x=w235, y=w234) -> (x+y=w233:cluster{dbl, dbl}[])
        n144 = call "PathToROI.vi"("Path In"=w233) -> ("ROI Out"=w240:T8)  [unwired: 10 in]
      }
      event Key Down {
        n145 = event-data() -> ("Char"=w245:i16)  [unwired: 1 in]
        n146 = property on="Path Drawer" class="ImageControl"() -> ("Last Mouse Position"=w244:cluster{"X":i32, "Y":i32})  [unwired: 2 in, 2 out]
        n147 = case shown="8" w245 {
          tunnel: w246 -> [w247 w256 _ _]
          tunnel: w241 -> [_ w255 w269 _]
          tunnel: w244 -> [_ w249 w270 _]
          tunnel: [w247 w248 w271 w288] -> w243
          tunnel: w242 -> [_ _ _ w288]
          frame 0, Default {
            # "Nothing"
          }
          frame 8 {
            # "If no nodes close to mouse do nothing"
            # "Backspace\nDelete node\nclosest to mouse"
            n148 = for {
              tunnel: w255 -> [w264] mode=indexing
              tunnel: [w263] -> w254 mode=indexing
              tunnel: w249 -> [w262]
              n149 = call "DistanceFormula.vi"("Point 2"=w262, "Point 1"=w264) -> ("Distance"=w263:dbl)  [unwired: 9 in]
            }
            n150 = Array Max & Min(array=w254) -> (min value=w252:dbl, min index (indices)=w253:i32)  [unwired: 2 out]
            n151 = Less?(x=w252, y=10.0) -> (x < y?=w250:bool)
            n152 = case shown="True" w250 {
              tunnel: w253 -> [_ w261]
              tunnel: w255 -> [_ w260]
              tunnel: w256 -> [w257 _]
              tunnel: [w257 w258] -> w248
              frame False {
              }
              frame True {
                n153 = Delete From Array(array=w260, index=w261) -> (array with subset deleted=w259:cluster{i32, i32}[])  [unwired: 1 in, 1 out]
                n154 = call "PathToROI.vi"("Path In"=w259) -> ("ROI Out"=w258:T8)  [unwired: 10 in]
              }
            }
          }
          frame 105 {
            # "Use math to find in between which points the mouse\nis hovering"
            # "I\nInsert node"
            n155 = Array Size(array=w269) -> (size(s)=w265:i32)
            n156 = for {
              N: w265 -> [_]
              tunnel: w269 -> [w287]
              tunnel: w270 -> [w284]
              tunnel: [w272] -> w267
              i -> [w272]
              stop <- w273 stop-if-true
              n157 = Index Array(array=w287, index #1=w272) -> (element #1=w286:cluster{i32, i32}, element #2=w285:cluster{i32, i32})  [unwired: 1 in]
              n158 = call "DistanceFormula.vi"("Point 2"=w285, "Point 1"=w286) -> ("Distance"=w283:dbl)  [unwired: 9 in]
              n159 = call "DistanceFormula.vi"("Point 2"=w284, "Point 1"=w286) -> ("Distance"=w282:dbl)  [unwired: 9 in]
              n160 = call "DistanceFormula.vi"("Point 2"=w284, "Point 1"=w285) -> ("Distance"=w281:dbl)  [unwired: 9 in]
              n161 = Square(x=w283) -> (x^2=w280:dbl)
              n162 = Square(x=w282) -> (x^2=w276:dbl)
              n163 = Square(x=w281) -> (x^2=w278:dbl)
              n164 = Add(x=w280, y=w276) -> (x+y=w279:dbl)
              n165 = Add(x=w280, y=w278) -> (x+y=w277:dbl)
              n166 = Greater Or Equal?(x=w279, y=w278) -> (x >= y?=w275:bool)
              n167 = Greater Or Equal?(x=w277, y=w276) -> (x >= y?=w274:bool)
              n168 = And(x=w275, y=w274) -> (x .and. y?=w273:bool)
            }
            n169 = Increment(x=w267) -> (x+1=w266:i32)
            n170 = Insert Into Array(array=w269, index=w266, new element=w270) -> (w268:cluster{i32, i32}[])
            n171 = call "PathToROI.vi"("Path In"=w268) -> ("ROI Out"=w271:T8)  [unwired: 10 in]
          }
          frame 122 {
            # "Restore last ROI"
            # "Z"
          }
        }
      }
      event "Path Drawer": Mouse Up {
        # "They have finished drawing a path, allow the event structure to run so\nthe starting point can snap at PathStorage can save the data"
        n172 = event-data() -> ()  [unwired: 1 in, 4 out]
      }
      event "LoadFromLocal": Value Change {
        # "Update Multiple Paths selector to reflect possible\nnew amount of paths in the editor"
        # "Update ROI on field image"
        # "Update PathStorage"
        # "Convert to array of PathFileDatas"
        # "Read string from file"
        # "Uses internal references to all the controls in this VI to update their values"
        n173 = event-data() -> ()  [unwired: 1 in, 2 out]
        n174 = local read "LocalFileNames"() -> (w300:string[])
        n175 = local read "LocalPaths"() -> (w301:i32)
        n176 = Current VI's Path() -> (path=w303:path)
        n177 = Strip Path(path=w303) -> (stripped path=w302:path)  [unwired: 1 out]
        n178 = Build Path(base path=w302, name or relative path="Paths") -> (appended path=w306:path)
        n179 = Index Array(array=w300, index=w301) -> (element=w305:string)
        n180 = Build Path(base path=w306, name or relative path=w305) -> (appended path=w304:path)
        n181 = Read from Text File(file (use dialog)=w304) -> (text=w307:string)  [unwired: 3 in, 3 out]
        n182 = Unflatten From JSON(JSON string=w307, type and defaults=T1[] []) -> (value=w289:T1[])  [unwired: 5 in, 1 out]
        "value" <- w289
        n183 = flat-sequence {
          frame #0 {
            n184 = Wait (ms)(milliseconds to wait=u32 100) -> ()  [unwired: 1 out]
          }
          frame #1 {
            n185 = local write "LoadFromLocal"(FALSE ("Export To File")) -> ()
          }
        }
        n186 = Index Array(array=w289) -> (element=w297:T1)  [unwired: 1 in]
        n187 = call "ClusterToControls.vi"("Path File Data"=w297) -> ("Path (px)"=w299:cluster{i32, i32}[])  [unwired: 10 in]
        n188 = Array Size(array=w289) -> (size(s)=w294:i32)
        n189 = property on="Multiple Paths" class="LstBox (strict)"("Number of Rows"=w294) -> (error out=w296:errorcluster)  [unwired: 2 in, 1 out]
        n190 = local write "PathsStorage"(w289) -> ()
        n191 = for {
          N: w294 -> [_]
          tunnel: [w310] -> w292 mode=indexing
          i -> [w311]
          n192 = Number To Decimal String(number=w311) -> (decimal integer string=w310:string)  [unwired: 1 in]
        }
        n193 = property on="Multiple Paths" class="LstBox (strict)"(error in=w296, "Item Names"=w292) -> (error out=w295:errorcluster)  [unwired: 1 in, 1 out]
        n194 = call "PathToROI.vi"("Path In"=w299) -> ("ROI Out"=w308:T8)  [unwired: 10 in]
        n195 = property on="Multiple Paths" class="LstBox (strict)"(error in=w295, "Size"=T7 {"Width"=92, "Height"=96}) -> (error out=w290:errorcluster)  [unwired: 1 in, 1 out]
        n196 = property on="Multiple Paths" class="LstBox (strict)"(error in=w290, "Value"=0 ("Active Row:Active Row Number")) -> ()  [unwired: 1 in, 2 out]
      }
      event "Flip Path": Value Change {
        # "Flip paths and update PathsStorage accordingly"
        # "Flip all the paths around the center of the field. \nOnly works if field syymetric, although if it is only close\nyou can edit the paths after flipping them."
        n197 = event-data() -> ()  [unwired: 1 in, 2 out]
        n198 = local read "Multiple Paths"() -> (w315:i32)
        n199 = local read "PathsStorage"() -> (w318:T1[])
        n200 = for {
          tunnel: w318 -> [w336] mode=indexing
          tunnel: [w331] -> w317 if=w324
          tunnel: [w328] -> w316 mode=indexing
          tunnel: w315 -> [w326]
          tunnel: [w325] -> w314 if=w324
          i -> [w327]
          w333 = cluster{i32, i32} {0, 191}
          # "Center of field"
          n201 = Unbundle By Name(w336) -> ("Meta.Path (px)"=w330:cluster{i32, i32}[], "Meta.StartingPositionPreset"=w320:u32)
          n202 = Equal?(x=w326, y=w327) -> (x = y?=w324:bool)
          n203 = Subtract(x=w330, y=w333) -> (x-y=w335:cluster{i32, i32}[])
          n204 = To Unsigned Word Integer(number=w320) -> (unsigned 16bit integer=w321:u16)
          n205 = Multiply(x=w335, y=cluster{i32, i32} {1, -1}) -> (x*y=w334:cluster{i32, i32}[])
          n206 = Type Cast(type=StartingPositions."1" ("StartingPosition"), x=w321) -> (*(type *) &x=w322:T3)
          n207 = Add(x=w334, y=w333) -> (x+y=w329:cluster{i32, i32}[])
          n208 = case shown="\"1\", Default" w322 {
            tunnel: [StartingPositions."3" ("StartingPosition") StartingPositions."2" ("StartingPosition") StartingPositions."1" ("StartingPosition") StartingPositions."5" ("StartingPosition") StartingPositions."4" ("StartingPosition") StartingPositions."No Preset" ("StartingPosition")] -> w325
            frame "1", Default {
            }
            frame "2" {
            }
            frame "3" {
            }
            frame "4" {
            }
            frame "5" {
            }
            frame "No Preset" {
            }
          }
          n209 = Bundle By Name(cluster=w336, "Meta.Path (px)"=w329, "Meta.StartingPositionPreset"=w325) -> (w328:T1)
          n210 = call "PathToROI.vi"("Path In"=w329) -> ("ROI Out"=w331:T8)  [unwired: 10 in]
        }
        n211 = local write "Flip Path"(FALSE ("Export To File")) -> ()
        n212 = local write "PathsStorage"(w316) -> ()
        n213 = local write "StartingPosition"(w314) -> ()
      }
      event "Multiple Paths": Value Change {
        # "Use references to controls on the front panel\nto update their values"
        # "Load the new path into the editor"
        n214 = event-data() -> ("NewVal"=w343:i32)  [unwired: 1 in, 5 out]
        n215 = local read "Multiple Paths"() -> (w345:i32)
        n216 = local read "PathsStorage"() -> (w346:T1[])
        n217 = Index Array(array=w346, index=w345) -> (element=w348:T1)
        n218 = call "ClusterToControls.vi"("Path File Data"=w348) -> ("Path (px)"=w347:cluster{i32, i32}[])  [unwired: 10 in]
        n219 = call "PathToROI.vi"("Path In"=w347) -> ("ROI Out"=w344:T8)  [unwired: 10 in]
      }
      event "Multiple Paths": Mouse Down? {
        # "2 for right click, 1 for regular click.\nBy turning double click into right click we open the options menu"
        n220 = event-data() -> ("Mods"=w354:cluster{"Double Click":bool, "Menu Key":bool})  [unwired: 1 in, 7 out]
        n221 = Unbundle By Name(w354) -> ("Double Click"=w353:bool)
        n222 = Select(t=u16 2 ("Button"), s=w353, f=u16 1) -> (s? t:f=w350:u16)
        n223 = local write "NoUpdate"(TRUE ("NoUpdate")) -> ()
        n224 = event-data("Button"=w350) -> ()  [unwired: 1 in, 1 out]
      }
      event "Multiple Paths": Shortcut Menu Selection (User) {
        # "Modify Paths Storage accordingly"
        n225 = event-data() -> ("ItemTag"=w359:string)  [unwired: 1 in, 7 out]
        n226 = local read "PathsStorage"() -> (w358:T1[])
        n227 = case shown="\"Clear Paths\"" w359 {
          tunnel: w358 -> [w362 w380 w414]
          tunnel: [w361 w385 w413] -> w357
          tunnel: w356 -> [_ _ _]
          tunnel: [_ w384 w405] -> w355
          frame "New Path", Default {
            # "Make the path a short line\nto start"
            # "Add a new path after the location they clicked"
            n228 = Array Size(array=w362) -> (size(s)=w368:i32)
            n229 = Increment(x=w368) -> (x+1=w375:i32)
            n230 = Decrement(x=w368) -> (x-1=w367:i32)
            n231 = Index Array(array=w362, index=w367) -> (element=w371:T1)
            n232 = Unbundle By Name(w371) -> ("Meta.Path (px)"=w370:cluster{i32, i32}[])
            n233 = for {
              N: w375 -> [_]
              tunnel: [w378] -> w377 mode=indexing
              i -> [w379]
              n234 = Number To Decimal String(number=w379) -> (decimal integer string=w378:string)  [unwired: 1 in]
            }
            n235 = property on="Multiple Paths" class="LstBox (strict)"("Number of Rows"=w375) -> (error out=w374:errorcluster)  [unwired: 2 in, 1 out]
            n236 = Reverse 1D Array(array=w370) -> (reversed array=w369:cluster{i32, i32}[])
            n237 = Index Array(array=w369) -> (element=w366:cluster{i32, i32})  [unwired: 1 in]
            n238 = Add(x=w366, y=cluster{i32, i32} {-60, 0}) -> (x+y=w364:cluster{i32, i32})
            n239 = property on="Multiple Paths" class="LstBox (strict)"(error in=w374, "Item Names"=w377) -> (error out=w373:errorcluster)  [unwired: 1 in, 1 out]
            n240 = Build Array(w366, w364) -> (w363:cluster{i32, i32}[])
            n241 = Bundle By Name(cluster=w371, "Meta.StartingPositionPreset"=StartingPositions."No Preset" ("StartingPosition"), "Meta.Path (px)"=w363) -> (w372:T1)
            n242 = Build Array (concatenate)(w362, w372) -> (w361:T1[])
            n243 = property on="Multiple Paths" class="LstBox (strict)"(error in=w373, "Size"=T7 {"Width"=92, "Height"=96}) -> ()  [unwired: 1 in, 2 out]
          }
          frame "Remove Path" {
            # "Don't remove\nif only one\nleft"
            n244 = Array Size(array=w380) -> (size(s)=w383:i32)
            n245 = Greater?(x=w383, y=1) -> (0:w381:bool)
            n246 = case shown="True" w381 {
              tunnel: [w386 w392] -> w385
              tunnel: [_ w391] -> w384
              tunnel: w380 -> [w386 w389]
              frame False {
              }
              frame True {
                # "Just load the first path in because I was lazy"
                # "Remove the path"
                n247 = local read "Multiple Paths"() -> (w388:i32)
                n248 = Delete From Array(array=w389, length=1, index=w388) -> (array with subset deleted=w392:T1[])  [unwired: 1 out]
                n249 = Index Array(array=w392) -> (element=w390:T1)  [unwired: 1 in]
                n250 = Array Size(array=w392) -> (size(s)=w395:i32)
                n251 = for {
                  N: w395 -> [_]
                  tunnel: [w401] -> w396 mode=indexing
                  i -> [w402]
                  n252 = Number To Decimal String(number=w402) -> (decimal integer string=w401:string)  [unwired: 1 in]
                }
                n253 = property on="Multiple Paths" class="LstBox (strict)"("Number of Rows"=w395) -> (error out=w398:errorcluster)  [unwired: 2 in, 1 out]
                n254 = call "ClusterToControls.vi"("Path File Data"=w390) -> ("Path (px)"=w393:cluster{i32, i32}[])  [unwired: 10 in]
                n255 = call "PathToROI.vi"("Path In"=w393) -> ("ROI Out"=w391:T8)  [unwired: 10 in]
                n256 = property on="Multiple Paths" class="LstBox (strict)"(error in=w398, "Item Names"=w396) -> (error out=w397:errorcluster)  [unwired: 1 in, 1 out]
                n257 = property on="Multiple Paths" class="LstBox (strict)"(error in=w397, "Size"=T7 {"Width"=92, "Height"=96}) -> (error out=w387:errorcluster)  [unwired: 1 in, 1 out]
                n258 = property on="Multiple Paths" class="LstBox (strict)"(error in=w387, "Value"=0 ("Active Row:Active Row Number")) -> ()  [unwired: 1 in, 2 out]
              }
            }
          }
          frame "Clear Paths" {
            w408 = u32 1 ("Number of Rows")
            # "Remove all but the first path"
            # "Keep only first path"
            n259 = for {
              N: w408 -> [_]
              tunnel: [w415] -> w412 mode=indexing
              i -> [w416]
              n260 = Number To Decimal String(number=w416) -> (decimal integer string=w415:string)  [unwired: 1 in]
            }
            n261 = property on="Multiple Paths" class="LstBox (strict)"("Number of Rows"=w408) -> (error out=w411:errorcluster)  [unwired: 2 in, 1 out]
            n262 = Index Array(array=w414) -> (element=w406:T1)  [unwired: 1 in]
            n263 = property on="Multiple Paths" class="LstBox (strict)"(error in=w411, "Item Names"=w412) -> (error out=w410:errorcluster)  [unwired: 1 in, 1 out]
            n264 = call "ClusterToControls.vi"("Path File Data"=w406) -> ("Path (px)"=w407:cluster{i32, i32}[])  [unwired: 10 in]
            n265 = property on="Multiple Paths" class="LstBox (strict)"(error in=w410, "Size"=T7 {"Width"=92, "Height"=96}) -> (error out=w404:errorcluster)  [unwired: 1 in, 1 out]
            n266 = call "PathToROI.vi"("Path In"=w407) -> ("ROI Out"=w405:T8)  [unwired: 10 in]
            n267 = property on="Multiple Paths" class="LstBox (strict)"(error in=w404, "Value"=0 ("Multiple Paths")) -> ()  [unwired: 1 in, 2 out]
            n268 = Build Array(w406) -> (w413:T1[])
          }
        }
        n269 = local write "PathsStorage"(w357) -> ()
      }
      event "SetStart": Value Change {
        # "Sets the start of the current selected path to the end of the previous one"
        n270 = event-data() -> ()  [unwired: 1 in, 6 out]
        n271 = local read "Multiple Paths"() -> (w419:i32)
        n272 = Not Equal To 0?(x=w419) -> (x != 0?=w420:bool)
        n273 = case shown="True" w420 {
          tunnel: w419 -> [_ w425]
          tunnel: [_ w421] -> w418
          tunnel: w417 -> [_ _]
          frame False {
          }
          frame True {
            n274 = Decrement(x=w425) -> (x-1=w434:i32)
            n275 = local read "PathsStorage"() -> (w424:T1[])
            n276 = Index Array(array=w424, index #1=w434, index #2=w425) -> (element #1=w433:T1, element #2=w427:T1)
            n277 = Unbundle By Name(w427) -> ("Meta.Path (px)"=w430:cluster{i32, i32}[])
            n278 = Unbundle By Name(w433) -> ("Meta.Path (px)"=w432:cluster{i32, i32}[])
            n279 = Reverse 1D Array(array=w432) -> (reversed array=w431:cluster{i32, i32}[])
            n280 = Index Array(array=w431) -> (element=w429:cluster{i32, i32})  [unwired: 1 in]
            n281 = Replace Array Subset(array=w430, new element=w429, index=0) -> (w422:cluster{i32, i32}[])
            n282 = Bundle By Name(cluster=w427, "Meta.Path (px)"=w422) -> (w426:T1)
            n283 = Replace Array Subset(array=w424, new element=w426, index=w425) -> (w423:T1[])
            n284 = local write "PathsStorage"(w423) -> ()
            n285 = call "PathToROI.vi"("Path In"=w422) -> ("ROI Out"=w421:T8)  [unwired: 10 in]
          }
        }
        n286 = flat-sequence {
          frame #0 {
            n287 = Wait (ms)(milliseconds to wait=u32 100) -> ()  [unwired: 1 out]
          }
          frame #1 {
            n288 = local write "SetStart"(FALSE ("SetStart")) -> ()
          }
        }
      }
    }
    n289 = Unbundle By Name(w56) -> ("Global Rectangle"=w70:i32[])
    n290 = Empty Array?(array=w70) -> (empty?=w54:bool)
    n291 = flat-sequence {
      tunnel: w46 -> [w88]
      tunnel: w49 -> [w89]
      tunnel: [w89] -> w48
      tunnel: [w88] -> w47
      tunnel: w48 -> [w93]
      tunnel: w47 -> [w92]
      frame #0 {
        n292 = Wait (ms)(milliseconds to wait=u32 40) -> ()  [unwired: 1 out]
      }
      frame #1 {
        # "Save all current info for the path (including params)"
        n293 = local read "PathsStorage"() -> (w94:T1[])
        n294 = local read "Points (px)"() -> (w100:cluster{dbl, dbl}[])
        n295 = local read "Multiple Paths"() -> (w96:i32)
        n296 = call "ControlsToCluster.vi"("Path (px)"=w100, "Path (in)"=w93) -> ("PathFileData"=w98:T1)  [unwired: 9 in]
        n297 = Array Size(array=w94) -> (size(s)=w95:i32)
        n298 = Less?(x=w96, y=w95) -> (x < y?=w99:bool)
        n299 = Empty Array?(array=w94) -> (empty?=w97:bool)
        n300 = case shown="False" w97 {
          tunnel: w96 -> [w106 _]
          tunnel: w99 -> [w105 _]
          tunnel: w98 -> [w104 w115]
          tunnel: w94 -> [w103 _]
          tunnel: [w102 w114] -> w90
          frame False {
            n301 = case shown="True" w105 {
              tunnel: w103 -> [w109 w113]
              tunnel: w104 -> [w108 w111]
              tunnel: w106 -> [_ w112]
              tunnel: [w107 w110] -> w102
              frame False {
                n302 = Build Array (concatenate)(w109, w108) -> (w107:T1[])
              }
              frame True {
                n303 = Replace Array Subset(array=w113, new element=w111, index=w112) -> (w110:T1[])
              }
            }
          }
          frame True {
            n304 = Build Array(w115) -> (w114:T1[])
          }
        }
        n305 = case shown="False" w92 {
          tunnel: w90 -> [w101 _]
          frame False {
            n306 = local write "PathsStorage"(w101) -> ()
          }
          frame True {
          }
        }
        n307 = local write "NoUpdate"(FALSE ("NoUpdate")) -> ()
      }
    }
  }
